vi "U8ArrayToHexString.vi"(11 "u8 Data[]":u8[](array[numeric]) format="%.0x") -> (3 "HEX String (0-9,A-F)":string)   [LabVIEW 2015, in "WZ5005E.lvlib"]
uses:
  WZ5005E.lvlib
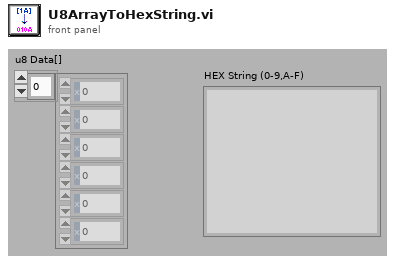
[diagram p1: front panel]
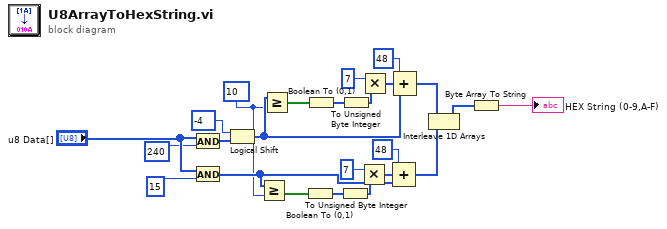
[diagram p0: block diagram]
diagram:
  w5 = u8 10
  n1 = And(x="u8 Data[]", y=u8 240) -> (x .and. y?=w3:u8[])
  n2 = And(x="u8 Data[]", y=u8 15) -> (x .and. y?=w21:u8[])
  n3 = Logical Shift(y=i8 -4, x=w3) -> (x << y=w12:u8[])
  n4 = Greater Or Equal?(x=w21, y=w5) -> (x >= y?=w20:bool[])
  n5 = Greater Or Equal?(x=w12, y=w5) -> (x >= y?=w11:bool[])
  n6 = Boolean To (0,1)(Boolean=w20) -> (0, 1=w18:i16[])
  n7 = Boolean To (0,1)(Boolean=w11) -> (0, 1=w6:i16[])
  n8 = To Unsigned Byte Integer(number=w18) -> (unsigned 8bit integer=w17:u8[])
  n9 = To Unsigned Byte Integer(number=w6) -> (unsigned 8bit integer=w7:u8[])
  n10 = Multiply(x=u8 7, y=w17) -> (x*y=w15:u8[])
  n11 = Multiply(x=u8 7, y=w7) -> (x*y=w9:u8[])
  n12 = Compound Arithmetic op=ADD(u8 48, w15, w21) -> (w22:u8[])
  n13 = Compound Arithmetic op=ADD(u8 48, w9, w12) -> (w13:u8[])
  n14 = Interleave 1D Arrays(w13, w22) -> (w14:u8[])
  n15 = Byte Array To String(unsigned byte array=w14) -> (string=→"HEX String (0-9,A-F)":string)
